vi "firmware 02 João Henrique Raduntz (1) (1).vi"() -> ()   [LabVIEW 2017]
uses:
  <vilib>/LabVIEW Interface for Arduino/Type Defs/Board Type.ctl
  <vilib>/LabVIEW Interface for Arduino/Type Defs/Connection Type.ctl
  <vilib>/LabVIEW Interface for Arduino/Type Defs/Pin Mode.ctl
  <vilib>/LabVIEW Interface for Arduino/LabVIEW Interface for Arduino.lvlib
panel:
  in  "stop":bool
  out "PEÇA ALTA":bool
  in  "SENSOR 3":bool
  out "PEÇA BAIXA":bool
  in  "SENSOR 1":bool
  in  "SENSOR 2":bool
  out "PEÇA DESCARTE":bool
  out "ESTEIRA":bool
  in  "LIGA MAQUINA":bool
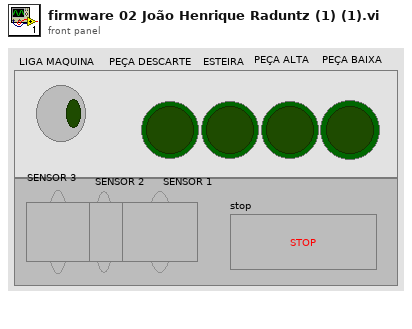
[diagram p1: front panel]
types:
  T1 = typedef "LabVIEW Interface for Arduino.lvlib/Pin Mode.ctl" = enum8{"Input", "Output"}
  T2 = typedef "LabVIEW Interface for Arduino.lvlib/Connection Type.ctl" = enum8{"USB / Serial", "XBEE", "BlueSmirf (Bluetooth)"}
  T3 = typedef "LabVIEW Interface for Arduino.lvlib/Board Type.ctl" = enum16{"Uno", "Dimuelanove w/Atmega 328", "Mega 2560"}
  T4 = typedef "LabVIEW Interface for Arduino.lvlib/Arduino Resource.ctl" = cluster{"VISA resource":refnum<visa-resource-name>, "Board Type":T3, "Connection Type":enum8{"USB / Serial"}, "Bytes Per Packet (15)":u8}
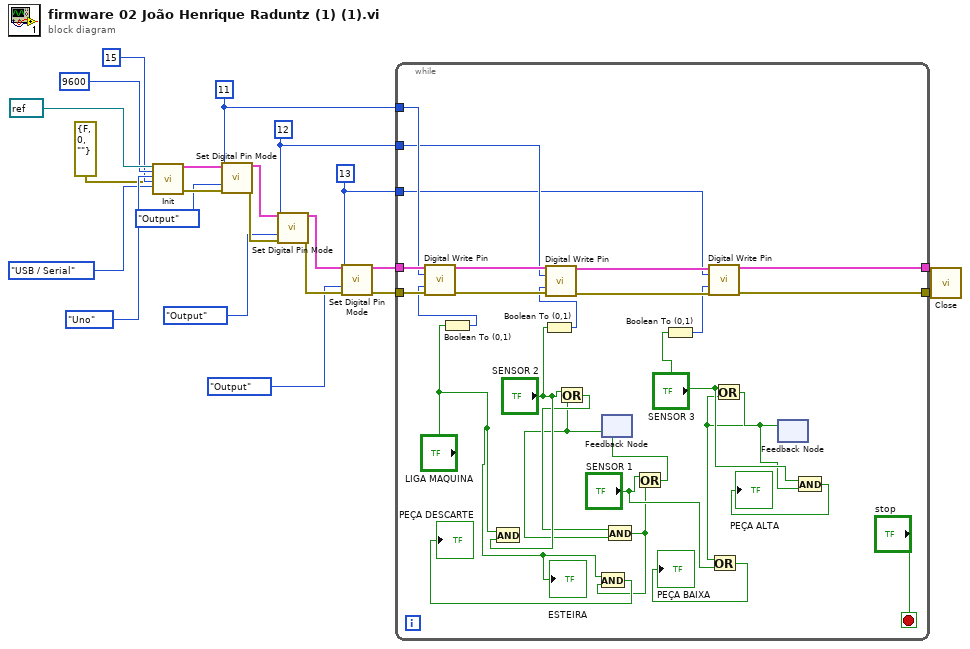
[diagram p0: block diagram]
diagram:
  w4 = u8 13 ("Digital I/O Pin")
  w5 = u8 12 ("Digital I/O Pin")
  w6 = u8 11 ("Digital I/O Pin")
  n1 = call <vilib>:"Init.vi"("VISA resource"=refnum<visa-resource-name> refnum, "Baud Rate (115200)"=u32 9600, "Board Type (Uno)"=Board_Type."Uno", "Bytes Per Packet (15)"=u32 15, "Connection Type (USB/Serial)"=Connection_Type."USB / Serial", "error in"=errorcluster {"status"=FALSE, "code"=0, "source"=""}) -> ("Arduino Resource"=w16:T4, "error out"=w13:errorcluster)  [unwired: 12 in]
  n2 = call <vilib>:"Set Digital Pin Mode.vi"("Arduino Resource"=w16, "Digital I/O Pin"=w6, "Pin Mode (Input)"=Pin_Mode."Output", "error in"=w13) -> ("Arduino Resource"=w15:T4, "error out"=w12:errorcluster)  [unwired: 10 in]
  n3 = call <vilib>:"Set Digital Pin Mode.vi"("Arduino Resource"=w15, "Digital I/O Pin"=w5, "Pin Mode (Input)"=Pin_Mode."Output", "error in"=w12) -> ("Arduino Resource"=w14:T4, "error out"=w11:errorcluster)  [unwired: 10 in]
  n4 = call <vilib>:"Set Digital Pin Mode.vi"("Arduino Resource"=w14, "Digital I/O Pin"=w4, "Pin Mode (Input)"=Pin_Mode."Output", "error in"=w11) -> ("Arduino Resource"=w10:T4, "error out"=w8:errorcluster)  [unwired: 10 in]
  n5 = while {
    tunnel: w10 -> [w50]
    tunnel: [w47] -> w9
    tunnel: w8 -> [w46]
    tunnel: [w43] -> w7
    tunnel: w6 -> [w42]
    tunnel: w5 -> [w41]
    tunnel: w4 -> [w40]
    stop <- "stop" stop-if-true
    n6 = Boolean To (0,1)(Boolean="LIGA MAQUINA") -> (0, 1=w38:i16)
    n7 = call <vilib>:"Digital Write Pin.vi"("Arduino Resource"=w50, "Digital I/O Pin (0)"=w42, "Value (0)"=w38, "error in"=w46) -> ("Arduino Resource"=w49:T4, "error out"=w45:errorcluster)  [unwired: 10 in]
    n8 = And(x="LIGA MAQUINA", y="SENSOR 2") -> ()  [unwired: 1 out]
    n9 = Boolean To (0,1)(Boolean="SENSOR 2") -> (0, 1=w37:i16)
    n10 = call <vilib>:"Digital Write Pin.vi"("Arduino Resource"=w49, "Digital I/O Pin (0)"=w41, "Value (0)"=w37, "error in"=w45) -> ("Arduino Resource"=w48:T4, "error out"=w44:errorcluster)  [unwired: 10 in]
    n11 = feedback #1() -> (w23:bool)  [unwired: 1 in]
    n12 = Or(x="SENSOR 2", y=w23) -> (x .or. y?=w25:bool)
    n13 = And(x=w25, y=w23) -> (x .and. y?=w27:bool)
    n14 = And(x="LIGA MAQUINA", y=w27) -> (x .and. y?=→"PEÇA DESCARTE":bool)
    n15 = Or(x="SENSOR 1", y=w27) -> (x .or. y?=w26:bool)
    n16 = feedback-in #1(w26) -> ()
    n17 = Boolean To (0,1)(Boolean="SENSOR 3") -> (0, 1=w36:i16)
    n18 = call <vilib>:"Digital Write Pin.vi"("Arduino Resource"=w48, "Digital I/O Pin (0)"=w40, "Value (0)"=w36, "error in"=w44) -> ("Arduino Resource"=w47:T4, "error out"=w43:errorcluster)  [unwired: 10 in]
    n19 = feedback #2() -> (w24:bool)  [unwired: 1 in]
    n20 = Or(x=w24, y="SENSOR 1") -> (x .or. y?=→"PEÇA BAIXA":bool)
    n21 = Or(x="SENSOR 3", y=w24) -> (x .or. y?=w28:bool)
    n22 = feedback-in #2(w28) -> ()
    n23 = And(x="SENSOR 3", y=w24) -> (x .and. y?=→"PEÇA ALTA":bool)
    "ESTEIRA" <- "LIGA MAQUINA"
  }
  n24 = call <vilib>:"Close.vi"("Arduino Resource"=w9, "error in"=w7) -> ()  [unwired: 13 in, 1 out]
